vi "draw_cross_section.vi"(7 "highlight?":bool, 8 "error in (no error)":errorcluster, 9 "depth":dbl[unit], 10 "Image.lvclass":refnum<class "Image.lvclass">, 11 "RoiGeneric in":refnum<class "RoiGeneric.lvclass">) -> (0 "error out":errorcluster, 3 "RoiGeneric out":refnum<class "RoiGeneric.lvclass">)   [LabVIEW 2010, in "RoiGeneric.lvclass"]
uses:
  RoiGeneric.lvclass
  common/classes/Image/Image/Image.lvclass
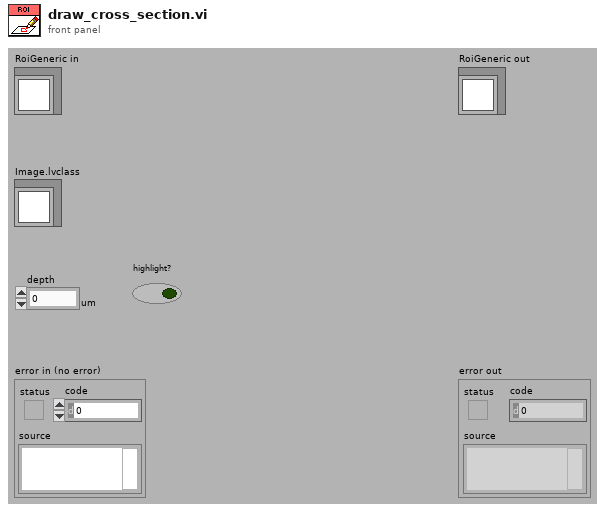
[diagram p1: front panel]
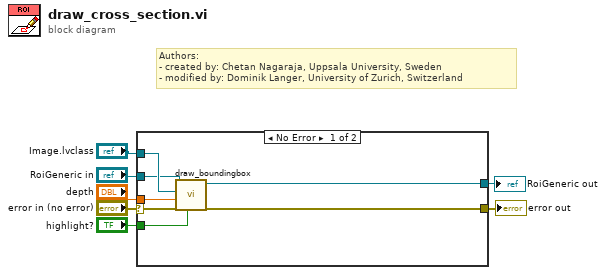
[diagram p0: block diagram]
diagram:
  # "Authors: \n- created by: Chetan Nagaraja, Uppsala University, Sweden\n- modified by: Dominik Langer, University of Zurich, Switzerland"
  n1 = case shown="No Error" "error in (no error)" {
    selector: "error in (no error)" -> [w14 w16]
    tunnel: [w13 w16] -> w6
    tunnel: [w9 w15] -> w4
    tunnel: "RoiGeneric in" -> [w10 w15]
    tunnel: "depth" -> [w12 _]
    tunnel: "Image.lvclass" -> [w11 _]
    tunnel: "highlight?" -> [w8 _]
    frame No Error {
      n2 = call-dynamic "draw_boundingbox.vi"("highlight?"=w8, "error in (no error)"=w14, "depth"=w12, "Image.lvclass"=w11, "RoiGeneric in"=w10) -> ("error out"=w13:errorcluster, "RoiGeneric out"=w9:refnum<class "RoiGeneric.lvclass">)  [unwired: 5 in]
    }
    frame Error {
    }
  }
  "error out" <- w6
  "RoiGeneric out" <- w4
